vi "ProgG_009_MG.vi"(1 "c":dbl=4.0, 2 "b":dbl=3.0, 3 "a":dbl=5.0) -> (0 "TAK - 1, NIE - 0":i32=1)   [LabVIEW 2021]
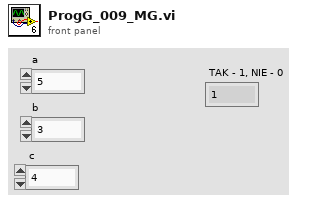
[diagram p1: front panel]
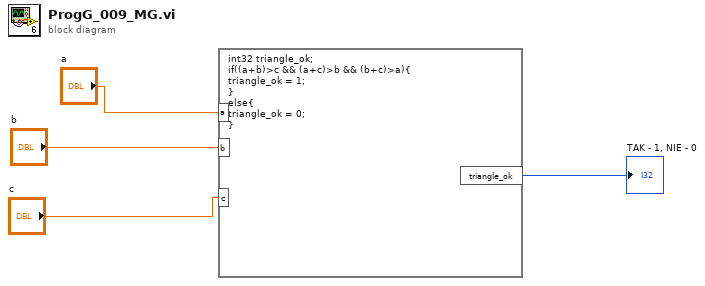
[diagram p0: block diagram]
diagram:
  n1 = formula code="int32 triangle_ok;\nif((a+b)>c && (a+c)>b && (b+c)>a){\ntriangle_ok = 1;\n}\nelse{\ntriangle_ok = 0;\n}"("a"="a", "b"="b", "c"="c") -> ("triangle_ok"=→"TAK - 1, NIE - 0":i32)
